vi "MainGUI.vi"(0 "reference in":refnum<class "JSONTextViewer.lvclass">, 5 "Error In":errorcluster) -> (14 "reference out":refnum<class "JSONTextViewer.lvclass">, 19 "Error Out":errorcluster)   [LabVIEW 2021, in "JSONTextViewer.lvlib" / "JSONTextViewer.lvclass"]
doc: "This template is based off of the Queued Message Handler design pattern and the Queued Message Handler project template that ships with LabVIEW.\n\nThe main difference is that the queue is private to this module and communication between modules is performed via Broadcast and Request events.\n\nRequest events are wrapped in public API methods and are handled in the Event Handling Loop (EHL) of this VI. Any module can register for Broadcast events sent by this module. The EHL generates messages based on user interface actions.\n\nThe Message Handling Loop (MHL) processes messages generated by the EHL, or by other messages. The messages are string values, so new messages can be added easily to the Message Cases case structure in the MHL. Each message cluster can also provide an optional value for Message Data, which is a variant that can be converted to whatever message-specific data is required.\n_____\nBased on Delacor QMH Project Template 4.2.0.63.\n\n<b>Note:</b> This VI was modified by the <b>Validate DQMH Module</b> tool to have the module name be passed as the Additional Information parameter with an Error Reported broadcast.\n\n<b>Note:</b> This VI was modified by the <b>Validate DQMH Module</b> tool to call the Release Message Queue VI in the top-level Error case."
uses:
  JSONTextViewer.lvclass
  JSONTextViewer_MessageData.ctl
  <vilib>/JDP Science/JSONtext/JSONtext.lvlib
panel:
  out "ID":string
  out "Last Command":string
  in  "Save":bool
  in  "JSON":string
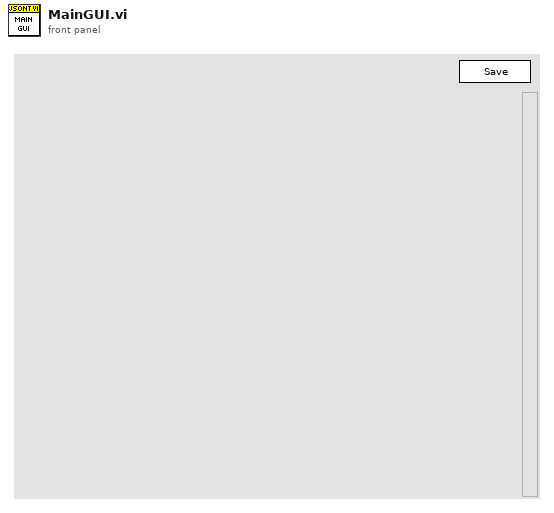
[diagram p1: front panel]
types:
  T1 = typedef "JSONTextViewer.lvlib/JSONTextViewer.lvclass/JSONTextViewer_MessageData.ctl" = cluster{"ShowWindow":cluster{"Send":cluster{"Show":bool}, "Receive":cluster{"Dummy":bool}}}
  T2 = cluster{"Event":refnum<event-registration>, "Command":string, "MessageData":T1, "ReplyQueue":refnum<queue>}
  T3 = cluster{"ReplyQueue":refnum<queue>, "Data":variant}
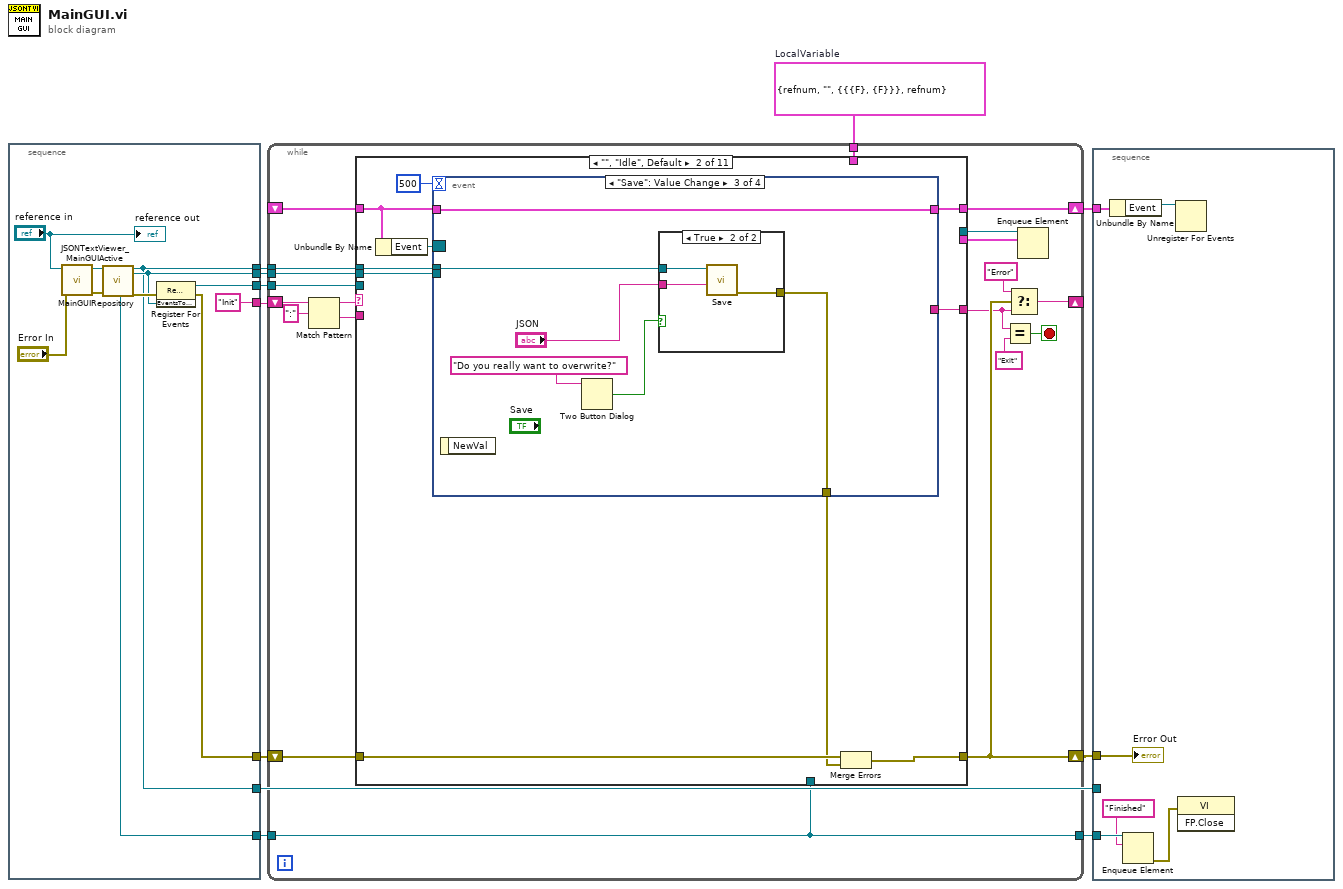
[diagram p0: block diagram]
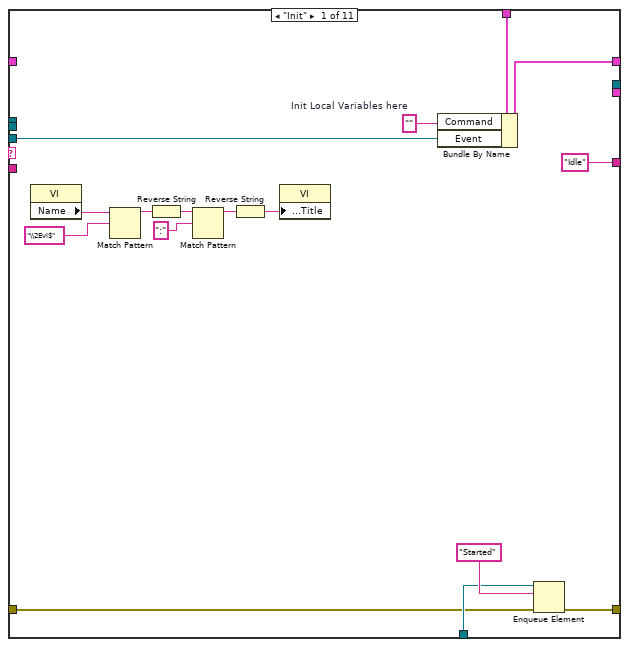
[diagram p2: hidden frame]
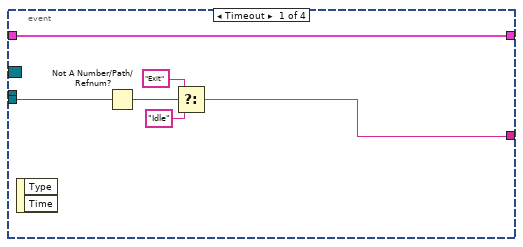
[diagram p3: hidden frame]
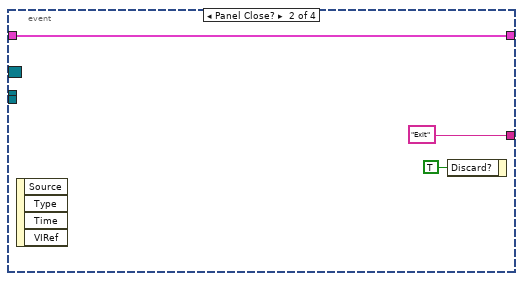
[diagram p4: hidden frame]
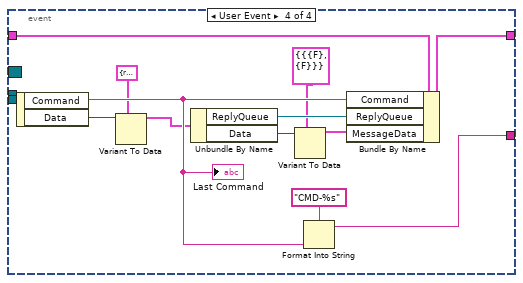
[diagram p6: hidden frame]
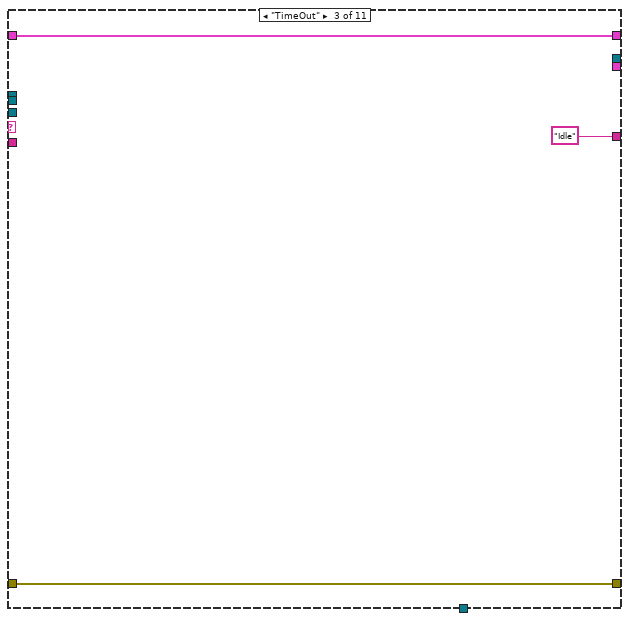
[diagram p7: hidden frame]
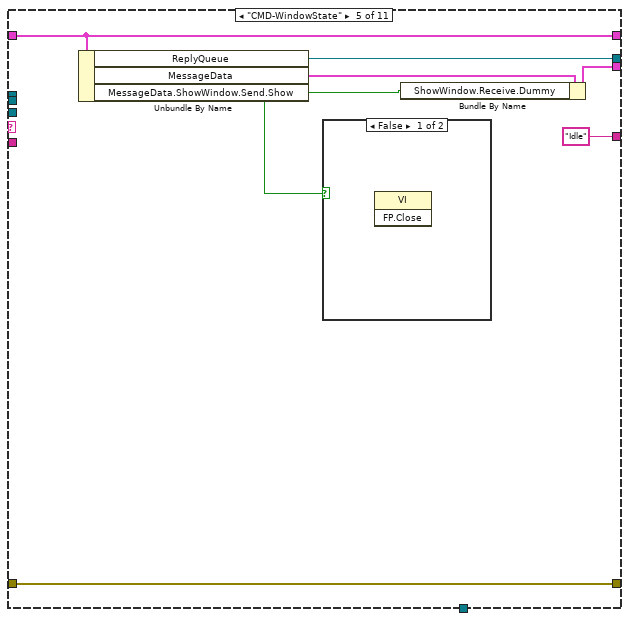
[diagram p9: hidden frame]
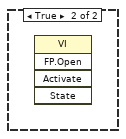
[diagram p10: hidden frame]
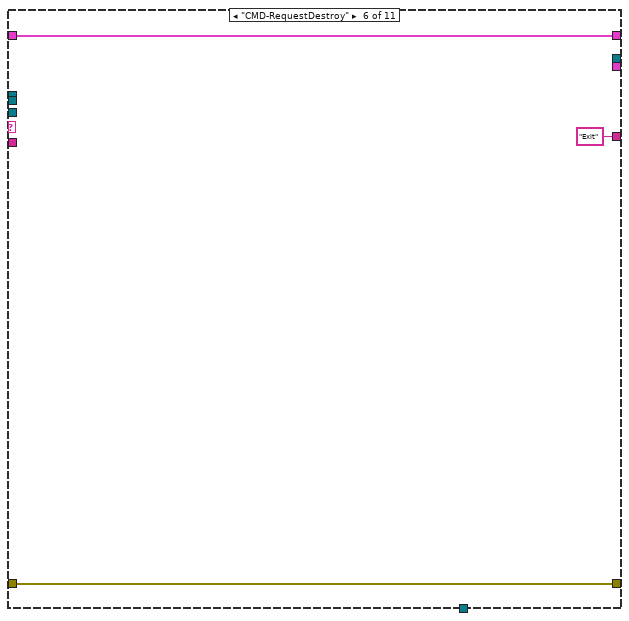
[diagram p11: hidden frame]
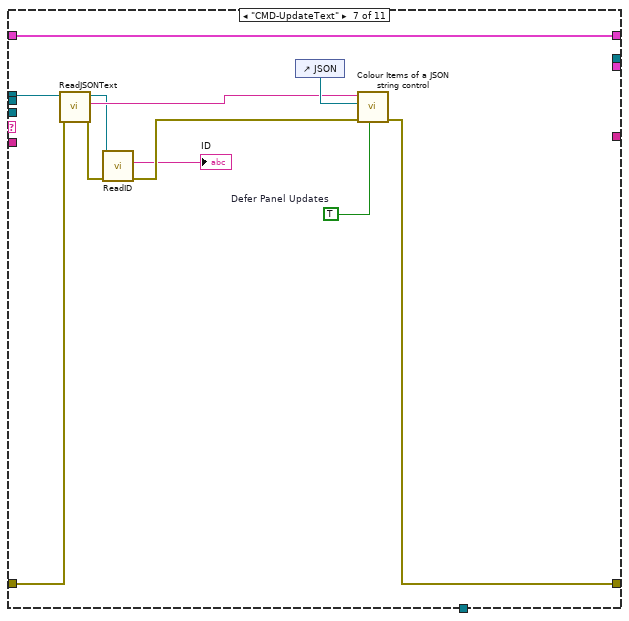
[diagram p12: hidden frame]
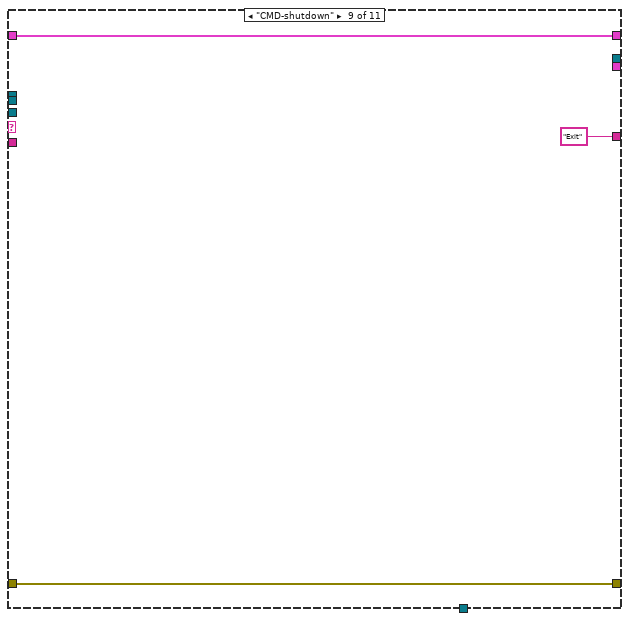
[diagram p14: hidden frame]
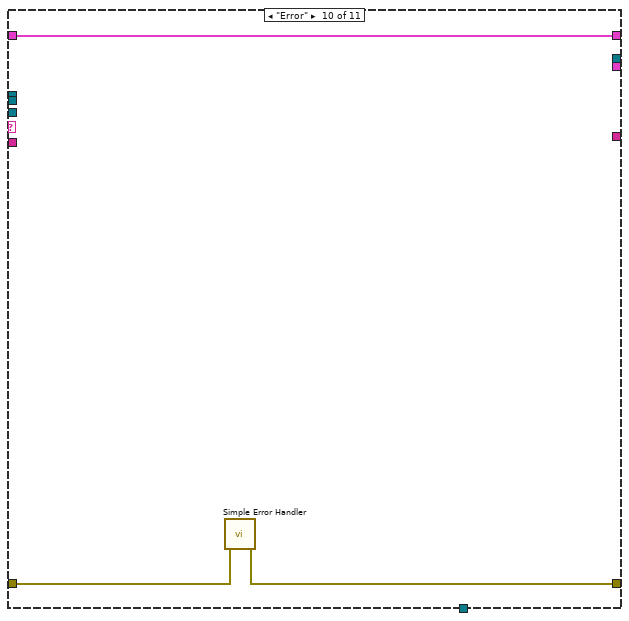
[diagram p15: hidden frame]
diagram:
  w6 = T2 {"Event"=refnum, "Command"="", "MessageData"={"ShowWindow"={"Send"={"Show"=FALSE}, "Receive"={"Dummy"=FALSE}}}, "ReplyQueue"=refnum}  # LocalVariable
  n1 = stacked-sequence {
    tunnel: [w17] -> w11
    tunnel: [w12] -> w9
    tunnel: [w20] -> w8
    tunnel: ["Init"] -> w7
    tunnel: [w18] -> w4
    tunnel: [w13] -> w2
    tunnel: [w12] -> w1
    frame #0 {
      n2 = call "JSONTextViewer_MainGUIActive.vi"("Error In"="Error In", "reference in"="reference in") -> ("Error Out"=w14:errorcluster, "reference out"=w16:refnum<class "JSONTextViewer.lvclass">)  [unwired: 8 in]
      n3 = call "MainGUIRepository.vi"("reference in"=w16, "Error In"=w14) -> ("ProcessSyncQueue"=w18:refnum<queue>, "reference out"=w12:refnum<class "JSONTextViewer.lvclass">, "EventsToProcess"=w13:refnum<user-event>, "Error Out"=w19:errorcluster)  [unwired: 10 in, 4 out]
      n4 = register-events(error in=w19, w13) -> (reference out=w20:refnum<event-registration>, error out=w17:errorcluster)  [unwired: 1 in]
      "reference out" <- "reference in"
    }
  }
  n5 = while {
    shift-right: [w35] -> w10
    shift-left: w11 -> [w40]
    tunnel: w9 -> [w41]
    tunnel: w8 -> [w42]
    shift-right: [w33] -> _
    shift-left: w7 -> [w38]
    shift-right: [w29] -> w5
    shift-left: _ -> [w28]
    tunnel: w6 -> [w27]
    tunnel: [w24] -> w3
    tunnel: w4 -> [w24]
    tunnel: w2 -> [w23]
    stop <- w30 stop-if-true
    n6 = Match Pattern(string=w38, regular expression=":") -> (before substring=w37:string, after substring=w36:string)  [unwired: 1 in, 2 out]
    n7 = case shown="\"\", \"Idle\", Default" w37 {
      tunnel: w40 -> [w43 w63 w101 w103 w110 w113 w120 w126 w129 w130 w134]
      tunnel: [w45 w60 w101 w103 w110 w113 w121 w126 w129 w131 w134] -> w35
      tunnel: w42 -> [w47 _ _ _ _ _ _ _ _ _ _]
      tunnel: w41 -> [_ w62 _ _ _ _ w118 _ _ _ _]
      tunnel: w36 -> [_ _ _ _ _ _ _ _ _ _ _]
      tunnel: ["Idle" ("t") w68 "Idle" ("t") _ "Idle" ("t") "Exit" ("y") _ _ "Exit" ("y") _ _] -> w32
      tunnel: [w58 w67 w99 w102 w108 w112 w124 w125 w127 w132 w133] -> w29
      tunnel: w28 -> [_ w66 w99 w102 w108 w112 w124 w125 w127 w132 w133]
      tunnel: w27 -> [w55 _ _ _ _ _ _ _ _ _ _]
      tunnel: [_ _ _ _ w107 _ _ _ _ _ _] -> w26
      tunnel: [_ _ _ _ w105 _ _ _ _ _ _] -> w25
      tunnel: w24 -> [w44 _ _ _ _ _ _ _ _ _ _]
      tunnel: w23 -> [_ w61 _ _ _ _ _ _ _ _ _]
      frame "Init" {
        w57 = ""  # Init Local Variables here
        n8 = property class="VI"() -> ("Name"=w54:string)  [unwired: 2 in, 2 out]
        n9 = Match Pattern(string=w54, regular expression="\\2Evi$") -> (before substring=w52:string)  [unwired: 1 in, 3 out]
        n10 = Reverse String(1:w52) -> (0:w51:string)
        n11 = Match Pattern(string=w51, regular expression=":") -> (before substring=w49:string)  [unwired: 1 in, 3 out]
        n12 = Reverse String(1:w49) -> (0:w48:string)
        n13 = property class="VI"("Front Panel.Title"=w48) -> ()  [unwired: 2 in, 2 out]
        n14 = Bundle By Name(cluster=w55, "Command"=w57, "Event"=w47) -> (w58:T2)
        n15 = Enqueue Element(queue=w44, element="Started", error in (no error)=w43) -> (error out=w45:errorcluster)  [unwired: 1 in, 2 out]
      }
      frame "", "Idle", Default {
        n16 = Unbundle By Name(w66) -> ("Event"=w65:refnum<event-registration>)
        n17 = event shown="[2] \"Save\": Value Change" {
          selector: w65 -> [_ _ _ _]
          dyn-events: _ -> [_ _ _ _]
          timeout: 500 -> [_ _ _ _]
          tunnel: [w69 "Exit" ("t") _ w95] -> w68
          tunnel: w66 -> [w74 w77 w83 w98]
          tunnel: [w74 w77 w83 w97] -> w67
          tunnel: w62 -> [_ _ w82 _]
          tunnel: w61 -> [w70 _ _ _]
          tunnel: [_ _ w81 _] -> w59
          event Timeout {
            n18 = event-data() -> ()  [unwired: 1 in, 2 out]
            n19 = Not A Number/Path/Refnum?(number/path/refnum=w70) -> (NaN/Path/Refnum?=w71:bool)
            n20 = Select(t="Exit", s=w71, f="Idle" ("t")) -> (s? t:f=w69:string)
          }
          event Panel Close? {
            n21 = event-data() -> ()  [unwired: 1 in, 4 out]
            n22 = event-data("Discard?"=TRUE) -> ()  [unwired: 1 in, 1 out]
          }
          event "Save": Value Change {
            n23 = event-data() -> ()  [unwired: 1 in, 1 out]
            n24 = Two Button Dialog(message="Do you really want to overwrite?") -> (T button?=w78:bool)  [unwired: 2 in]
            n25 = case shown="True" w78 {
              tunnel: w82 -> [_ w86]
              tunnel: [_ w85] -> w81
              tunnel: "JSON" -> [_ w84]
              frame False {
              }
              frame True {
                n26 = call-dynamic "Save.vi"("Text"=w84, "reference in"=w86) -> ("Error Out"=w85:errorcluster)  [unwired: 8 in, 1 out]
              }
            }
          }
          event User Event {
            n27 = event-data() -> ("Command"=w94:string, "Data"=w93:variant)  [unwired: 1 in]
            "Last Command" <- w94
            n28 = Variant To Data(type=T3 {"ReplyQueue"=refnum, "Data"=variant} ("output cluster"), Variant=w93) -> (data=w91:T3)  [unwired: 1 in, 1 out]
            n29 = Unbundle By Name(w91) -> ("ReplyQueue"=w90:refnum<queue>, "Data"=w89:variant)
            n30 = Variant To Data(type=T1 {"ShowWindow"={"Send"={"Show"=FALSE}, "Receive"={"Dummy"=FALSE}}} ("MessageData"), Variant=w89) -> (data=w88:T1)  [unwired: 1 in, 1 out]
            n31 = Format Into String(format string="CMD-%s", w94) -> (resulting string=w95:string)  [unwired: 2 in, 1 out]
            n32 = Bundle By Name(cluster=w98, "Command"=w94, "ReplyQueue"=w90, "MessageData"=w88) -> (w97:T2)
          }
        }
        n33 = Merge Errors(w63, w59) -> (w60:errorcluster)
      }
      frame "TimeOut" {
      }
      frame "---- COMMANDS START----" {
      }
      frame "CMD-WindowState" {
        n34 = Unbundle By Name(w108) -> ("ReplyQueue"=w107:refnum<queue>, "MessageData"=w106:T1, "MessageData.ShowWindow.Send.Show"=w104:bool)
        n35 = case shown="False" w104 {
          frame False {
            n36 = invoke class="VI" method="FP.Close"() -> ()  [unwired: 3 in, 3 out]
          }
          frame True {
            n37 = invoke class="VI" method="FP.Open"() -> ()  [unwired: 5 in, 5 out]
          }
        }
        n38 = Bundle By Name(cluster=w106, "ShowWindow.Receive.Dummy"=w104) -> (w105:T1)
      }
      frame "CMD-RequestDestroy" {
      }
      frame "CMD-UpdateText" {
        w123 = TRUE  # Defer Panel Updates
        n39 = call-dynamic "ReadJSONText.vi"("Error In"=w120, "reference in"=w118) -> ("Error Out"=w117:errorcluster, "JSONText"=w119:string, "reference in"=w116:refnum<class "JSONTextViewer.lvclass">)  [unwired: 7 in]
        n40 = call-dynamic "ReadID.vi"("Error In"=w117, "reference in"=w116) -> ("Error Out"=w115:errorcluster, "ID"=→"ID":string)  [unwired: 7 in, 1 out]
        n41 = control-ref of="JSON"() -> (w122:refnum<vi>)
        n42 = call <vilib>:"Colour Items of a JSON string control.vi"("Defer Panel Updates"=w123, "error in (no error)"=w115, "String Control"=w122, "JSON"=w119) -> ("error out"=w121:errorcluster)  [unwired: 7 in]
      }
      frame "----- COMMANDS END ----" {
      }
      frame "CMD-shutdown" {
      }
      frame "Error" {
        n43 = call <vilib>:"Simple Error Handler.vi"("error in (no error)"=w130) -> ("error out"=w131:errorcluster)  [unwired: 4 in, 4 out]
      }
      frame "----- UI ACTIONS -----" {
      }
    }
    n44 = Equal?(x=w32, y="Exit") -> (x = y?=w30:bool)
    n45 = Select(t="Error", s=w35, f=w32) -> (s? t:f=w33:string)
    n46 = Enqueue Element(queue=w26, element=w25) -> ()  [unwired: 2 in, 3 out]
  }
  n47 = stacked-sequence {
    tunnel: w10 -> [w140]
    tunnel: w3 -> [w137]
    tunnel: w5 -> [w139]
    tunnel: w1 -> [_]
    frame #0 {
      n48 = Unbundle By Name(w139) -> ("Event"=w138:refnum<event-registration>)
      n49 = Enqueue Element(queue=w137, element="Finished") -> (error out=w136:errorcluster)  [unwired: 2 in, 2 out]
      n50 = Unregister For Events(event registration refnum=w138) -> ()  [unwired: 1 in, 1 out]
      n51 = invoke class="VI" method="FP.Close"(error in=w136) -> ()  [unwired: 2 in, 3 out]
      "Error Out" <- w140
    }
  }
